vi "AO_benchmarking.vi"() -> ()   [LabVIEW 2020]
uses:
  <vilib>/rvi/Emulation/niFpgaGetClockAttributes.vi
  <vilib>/rvi/Emulation/niFpgaSctlEmulationGetInTimedLoop.vi
  <vilib>/rvi/Emulation/niFpgaEmulationReportErrorSimple.vi
  <vilib>/rvi/eio/common/nirviEmuTemplateMethod_errors.vi
  <vilib>/rvi/Emulation/niFpgaCriticalErrorInLSC.vi
  <vilib>/eio/EIONode/EIONode.xnode
panel:
  out "AO Loop time [ticks] 2":u32
  out "AO Loop time [ticks]":u32
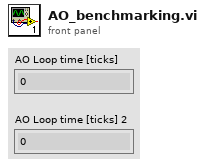
[diagram p1: front panel]
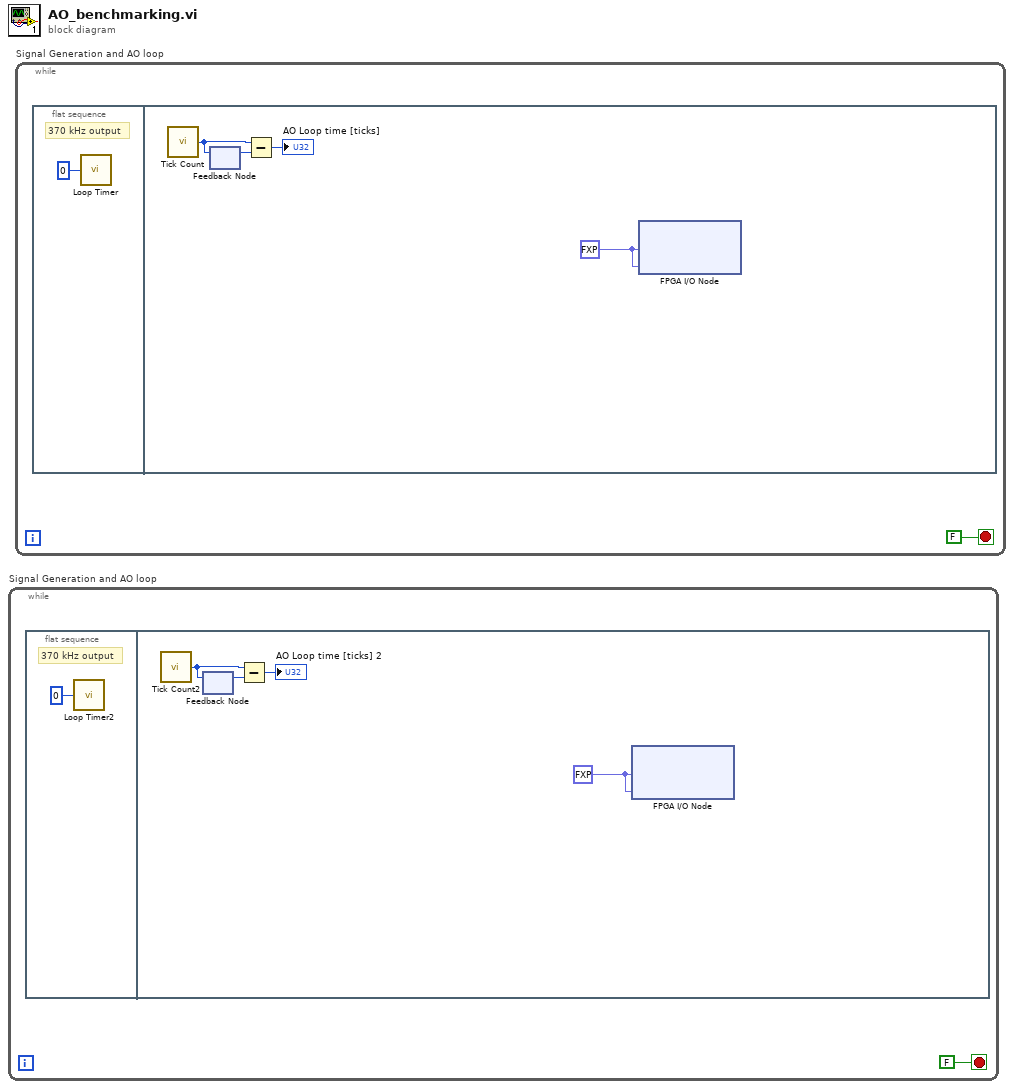
[diagram p0: block diagram]
diagram:
  n1 = while "Signal Generation and AO loop" {
    stop <- FALSE stop-if-true
    n2 = flat-sequence {
      frame #0 {
        # "370 kHz output"
        n3 = call "Loop Timer2"("Count(Ticks)"=u32 0) -> ()  [unwired: 1 out]
      }
      frame #1 {
        w3 = fxp<+/-,20,5> 0.0 ("Mod3/AO0")
        n4 = call "Tick Count2"() -> ("Tick Count(Ticks)"=w6:u32)
        n5 = feedback #1() -> (w5:u32)  [unwired: 1 in]
        n6 = feedback-in #1(w6) -> ()
        n7 = Subtract(x=w6, y=w5) -> (x-y=→"AO Loop time [ticks] 2":u32)
        n8 = xnode "FPGA I/O Node"("Mod4/AO0"=w3, "Mod4/AO1"=w3) -> ()  [unwired: 2 in, 2 out]
      }
    }
  }
  n9 = while "Signal Generation and AO loop" {
    stop <- FALSE stop-if-true
    n10 = flat-sequence {
      frame #0 {
        # "370 kHz output"
        n11 = call "Loop Timer"("Count(Ticks)"=u32 0) -> ()  [unwired: 1 out]
      }
      frame #1 {
        w9 = fxp<+/-,20,5> 0.0 ("Mod3/AO0")
        n12 = call "Tick Count"() -> ("Tick Count(Ticks)"=w12:u32)
        n13 = feedback #2() -> (w11:u32)  [unwired: 1 in]
        n14 = feedback-in #2(w12) -> ()
        n15 = Subtract(x=w12, y=w11) -> (x-y=→"AO Loop time [ticks]":u32)
        n16 = xnode "FPGA I/O Node"("Mod3/AO0"=w9, "Mod3/AO1"=w9) -> ()  [unwired: 2 in, 2 out]
      }
    }
  }
